vi "Simulated_Robot_Globals.vi"() -> ()   [LabVIEW 2019]
uses:
  DiffDriveSim/DiffDriveSim_EncoderValues.ctl
  <vilib>/Rock Robotics/WPI/Simulation/Protocol/Devices/Encoder/Encoder proto.ctl
  <vilib>/Rock Robotics/WPI/Simulation/Protocol/Devices/Encoder/Encoder data protoo.ctl
  <vilib>/Rock Robotics/WPI/Simulation/Protocol/Devices/Gyro/Gyro proto.ctl
  <vilib>/Rock Robotics/WPI/Simulation/Protocol/Devices/Gyro/Gyro Data proto.ctl
  <vilib>/Rock Robotics/WPI/ThirdParty/JAS_Junk/TrajLib/TypeDef/DIFF_DRIVE_TRAIN_SIM.ctl
  <vilib>/Rock Robotics/WPI/ThirdParty/JAS_Junk/TrajLib/TypeDef/LINEAR_SYSTEM.ctl
  <vilib>/Analysis/Matrix/Datatypes/RealMatrix.ctl
  <vilib>/Rock Robotics/WPI/ThirdParty/JAS_Junk/TrajLib/TypeDef/DCMOTOR.CTL
  <vilib>/Rock Robotics/WPI/Simulation/Protocol/Devices/PWM/PWM proto.ctl
  <vilib>/Rock Robotics/WPI/Simulation/Protocol/Devices/PWM/PWM data proto.ctl
  <vilib>/Analysis/Matrix/NI_Matrix.lvlib
  <vilib>/Rock Robotics/WPI/ThirdParty/JAS_Junk/TrajLib/Trajectory_Library.lvlib
  <vilib>/Rock Robotics/WPI/ThirdParty/JAS_Junk/TrajLib/TypeDef/TRANSLATION2D.ctl
  <vilib>/Rock Robotics/WPI/ThirdParty/JAS_Junk/TrajLib/TypeDef/ROTATION2D.ctl
  <vilib>/Rock Robotics/WPI/ThirdParty/JAS_Junk/TrajLib/TypeDef/POSE2D.ctl
panel:
  out "Simulation Running":bool
  in  "Initial Robot Pose":T1={"TRANSLATION"={"X"=0.0, "Y"=0.0}, "ROTATION"={"VALUE"=0.0, "COS"=1.0, "SIN"=0.0}} {"ROTATION"."SIN" format="%13.4f"; "ROTATION"."COS" format="%13.4f"; "ROTATION"."VALUE" format="%13.4f"; "TRANSLATION"."Y" format="%14.3f"; "TRANSLATION"."X" format="%14.3f"}
  out "PWM 1 Data":T4
  out "PWM  0 Data":T4
  out "Gyro Value":dbl
  out "DiffDriveTrainSim":T6 {"m_Motor"."Jr_KgM2" format="%13.5p"; "m_Motor"."L_H" format="%13.5p"; "m_Motor"."Kt_NMPerAmp" format="%13.5p"; "m_Motor"."KvINV_RadPerSecPerVolt" format="%13.5p"; "m_Motor"."R_Ohms" format="%13.5p"; "m_Motor"."FreeSpeed_RadPerSec" format="%13.5p"; "m_Motor"."FreeCurrent_Amps" format="%13.5p"; "m_Motor"."StallCurrent_Amps" format="%13.5p"; "m_Motor"."StallTorque_NM" format="%13.5p"; "m_Motor"."nominalVoltage_Volts" format="%13.5p"}
  out "Gyro":T10
  out "Enc Left":T12={"type"="Encoder", "device"="", "name"="", "data"={"<init"=FALSE, ">count"=0.0, ">period"=0.0, "<samples_to_avg"=0, "<offset"=0.0, "<channel_a"=0, "<channel_b"=0}}
  out "Enc Right":T12={"type"="Encoder", "device"="", "name"="", "data"={"<init"=FALSE, ">count"=0.0, ">period"=0.0, "<samples_to_avg"=0, "<offset"=0.0, "<channel_a"=0, "<channel_b"=0}}
  out "Right Encoder Values":T14
  out "Left Encoder Values":T14
  out "Ctrl Loop Offset MS":dbl
  out "Restart":bool
  out "Battery Current":dbl
  out "Battery Voltage":dbl
  out "PWM 1":dbl
  out "PWM 0":dbl
  out "Robot Enabled":bool
  # "<States, 1>"
  # "<Outputs, 1>"
  # "<Inputs, 1>"
  # "<Outputs, 1>"
  # "<States,States>"
  # "<States,Inputs>"
  # "<Outputs,States>"
  # "<Outputs,Inputs>"
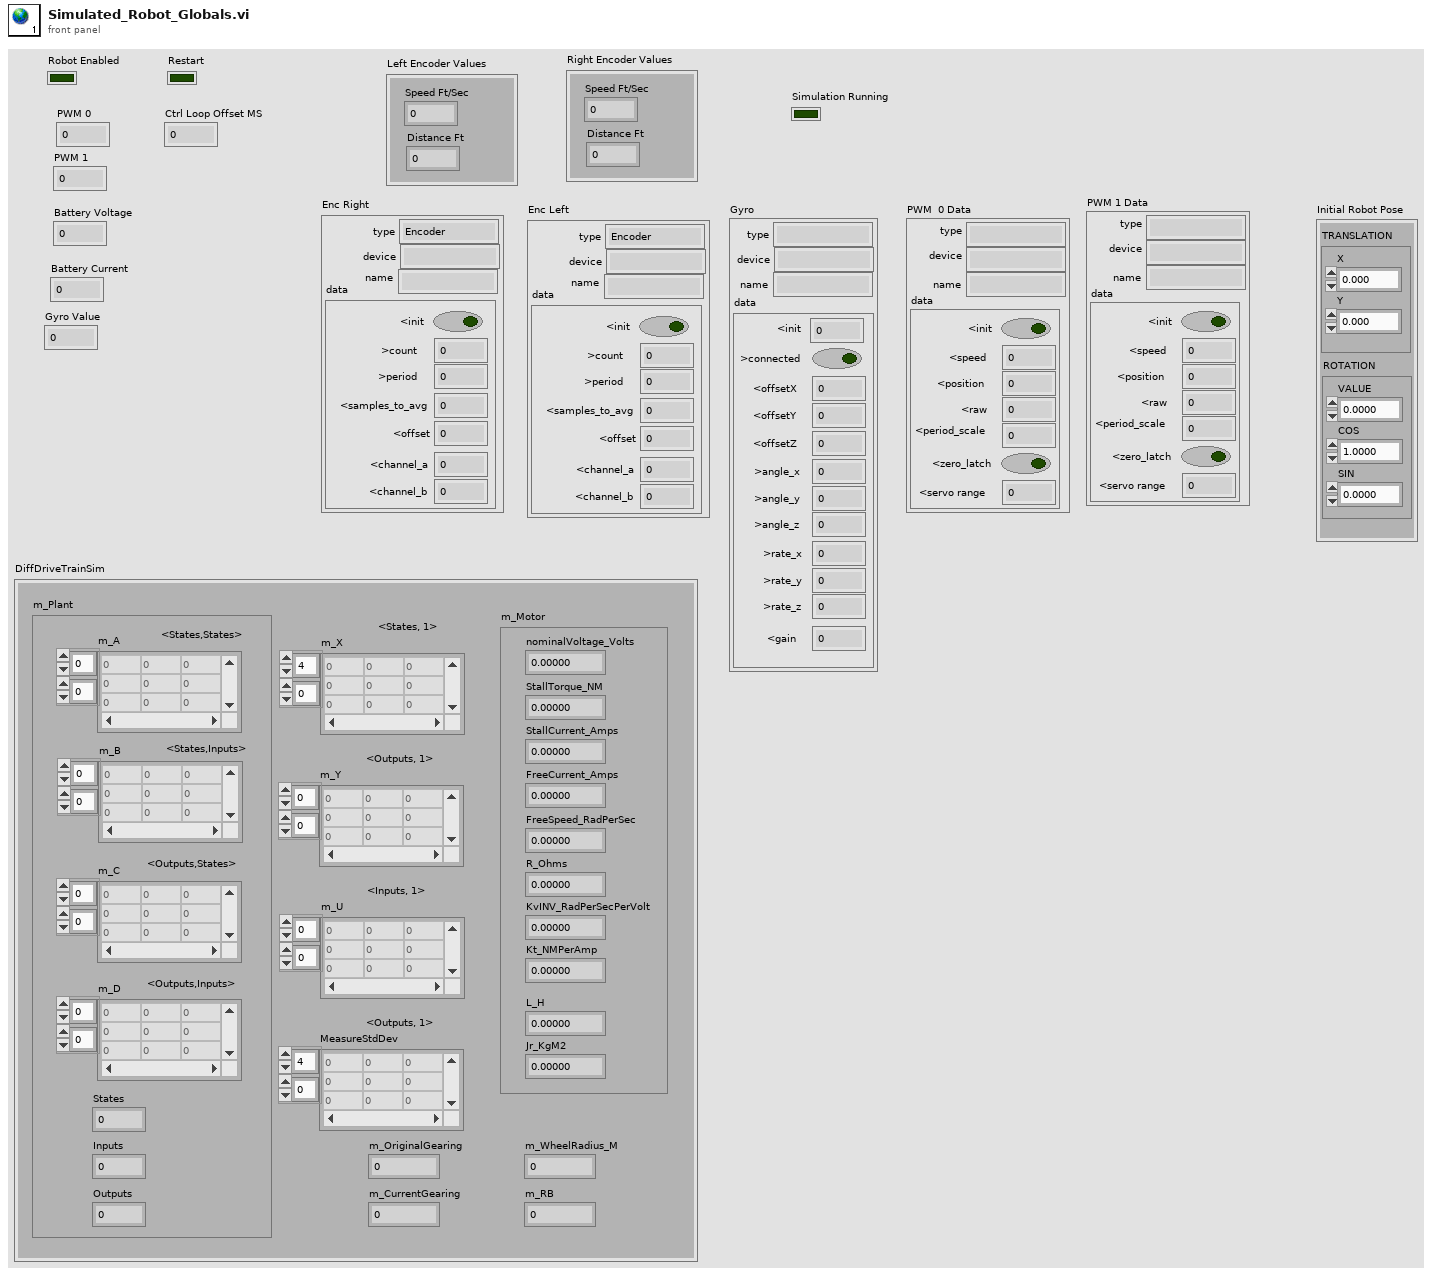
[diagram p1: front panel]
types:
  T1 = typedef "Trajectory_Library.lvlib/POSE2D.ctl" = cluster{"TRANSLATION":T2, "ROTATION":T3}
  T2 = typedef "Trajectory_Library.lvlib/TRANSLATION2D.ctl" = cluster{"X":dbl, "Y":dbl}
  T3 = typedef "Trajectory_Library.lvlib/ROTATION2D.ctl" = cluster{"VALUE":dbl, "COS":dbl, "SIN":dbl}
  T4 = typedef "PWM proto.ctl" = cluster{"type":string, "device":string, "name":string, "data":T5}
  T5 = typedef "PWM data proto.ctl" = cluster{"<init":bool, "<speed":dbl, "<position":dbl, "<raw":dbl, "<period_scale":dbl, "<zero_latch":bool, "<servo range":dbl}
  T6 = typedef "Trajectory_Library.lvlib/DIFF_DRIVE_TRAIN_SIM.ctl" = cluster{"m_Plant":T7, "m_X":T8, "m_Y":T8, "m_U":T8, "MeasureStdDev":T8, "m_Motor":T9, "m_OriginalGearing":dbl, "m_CurrentGearing":dbl, "m_WheelRadius_M":dbl, "m_RB":dbl}
  T7 = typedef "Trajectory_Library.lvlib/LINEAR_SYSTEM.ctl" = cluster{"m_A":T8, "m_B":T8, "m_C":T8, "m_D":T8, "States":i32, "Inputs":i32, "Outputs":i32}
  T8 = typedef "NI_Matrix.lvlib/RealMatrix.ctl" = dbl[][]
  T9 = typedef "Trajectory_Library.lvlib/DCMOTOR.CTL" = cluster{"nominalVoltage_Volts":dbl, "StallTorque_NM":dbl, "StallCurrent_Amps":dbl, "FreeCurrent_Amps":dbl, "FreeSpeed_RadPerSec":dbl, "R_Ohms":dbl, "KvINV_RadPerSecPerVolt":dbl, "Kt_NMPerAmp":dbl, "L_H":dbl, "Jr_KgM2":dbl}
  T10 = typedef "Gyro proto.ctl" = cluster{"type":string, "device":string, "name":string, "data":T11}
  T11 = typedef "Gyro Data proto.ctl" = cluster{"<init":i32, ">connected":bool, "<offsetX":dbl, "<offsetY":dbl, "<offsetZ":dbl, ">angle_x":dbl, ">angle_y":dbl, ">angle_z":dbl, ">rate_x":dbl, ">rate_y":dbl, ">rate_z":dbl, "<gain":dbl}
  T12 = typedef "Encoder proto.ctl" = cluster{"type":string, "device":string, "name":string, "data":T13}
  T13 = typedef "Encoder data protoo.ctl" = cluster{"<init":bool, ">count":dbl, ">period":dbl, "<samples_to_avg":i32, "<offset":dbl, "<channel_a":i32, "<channel_b":i32}
  T14 = typedef "DiffDriveSim_EncoderValues.ctl" = cluster{"Speed Ft/Sec":dbl, "Distance Ft":dbl}
diagram:
